vi "G#Debugger_OpenAttributeReference.vi"(0 "vi path":path, 5 "error in (no error)":errorcluster) -> (14 "vi reference":refnum<vi>, 19 "error out":errorcluster)   [LabVIEW 2017, in "G#Debugger.lvlib"]
uses:
  <vilib>/addons/_AddQ/G#Debugger/G#Debugger.lvlib
  <vilib>/Utility/miscctls.llb/LVPointTypeDef.ctl
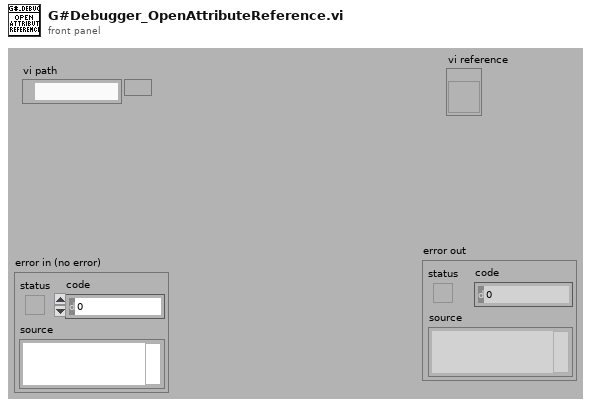
[diagram p1: front panel]
types:
  T1 = enum32{"invalid VI type", "Standard VI", "Control VI", "Global VI", "Polymorphic VI", "Configuration VI", "SubSystem", "Facade VI", "Method VI", "Statechart Diagram VI"}
  T2 = typedef "LVPointTypeDef.ctl" = cluster{"Horizontal":i16, "Vertical":i16}
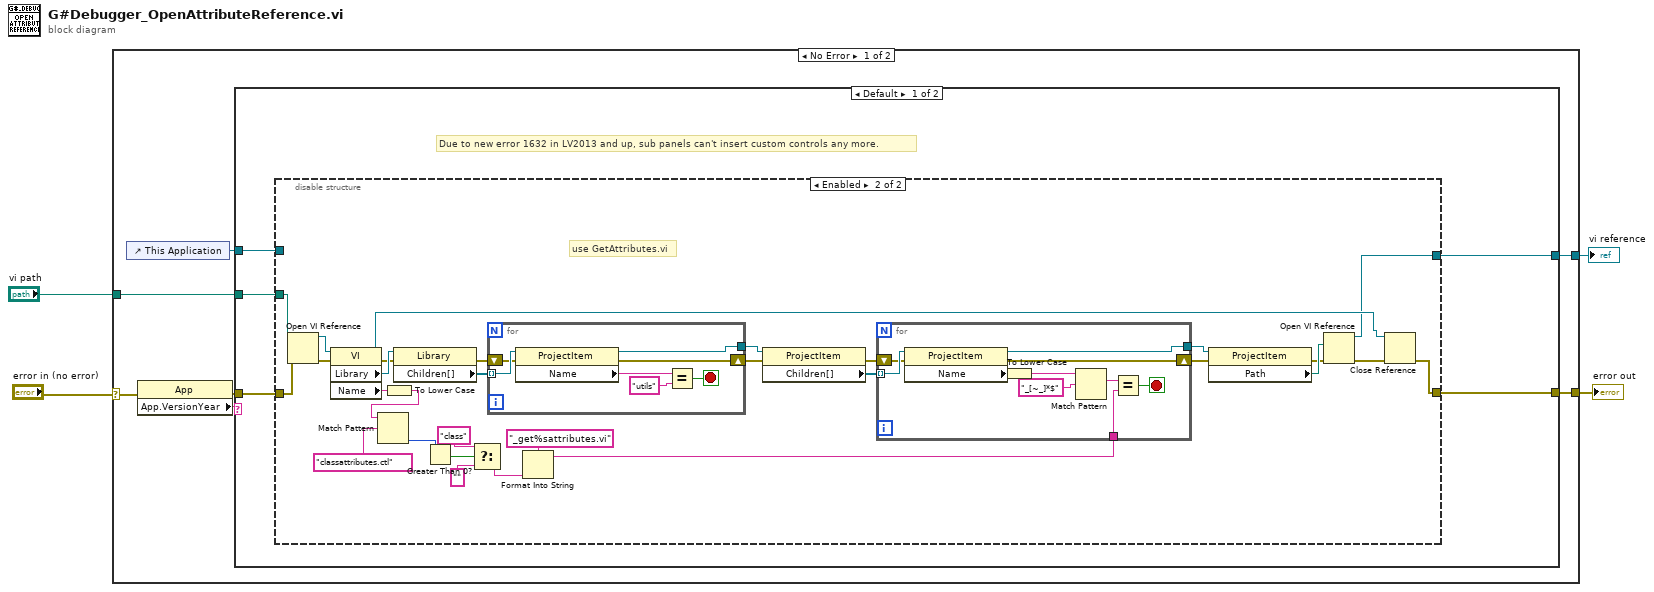
[diagram p0: block diagram]
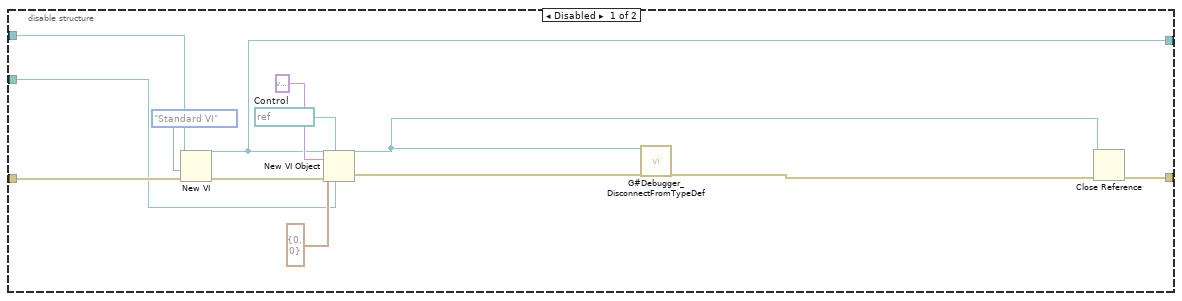
[diagram p2: hidden frame]
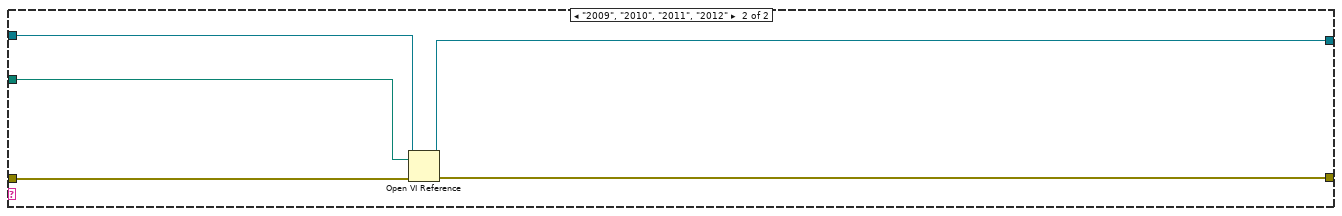
[diagram p3: hidden frame]
diagram:
  n1 = case shown="No Error" "error in (no error)" {
    selector: "error in (no error)" -> [w7 w82]
    tunnel: "vi path" -> [w9 _]
    tunnel: [w8 w82] -> w2
    tunnel: [w5 _] -> w3
    frame No Error {
      n2 = control-ref of="This Application"() -> (w6:refnum<vi>)
      n3 = property class="App"(error in=w7) -> (error out=w10:errorcluster, "App.VersionYear"=w11:string)  [unwired: 1 in, 1 out]
      n4 = case shown="Default" w11 {
        tunnel: w10 -> [w16 w81]
        tunnel: w9 -> [w14 w80]
        tunnel: [w15 w79] -> w8
        tunnel: w6 -> [w13 w78]
        tunnel: [w12 w77] -> w5
        frame Default {
          # "Due to new error 1632 in LV2013 and up, sub panels can't insert custom controls any more."
          n5 = disable-structure shown="Enabled" {
            disable-tunnel: w16 -> [w26 w45]
            disable-tunnel: [w25 w41] -> w15
            disable-tunnel: w14 -> [w24 w44]
            disable-tunnel: w13 -> [w22 _]
            disable-tunnel: [w20 w40] -> w12
            frame Disabled {
              w29 = refnum<vi> refnum  # Control
              n6 = New VI(8:w26, 9:T1."Standard VI" ("vi type (standard vi)"), 11:w22) -> (0:w23:errorcluster, 3:w20:refnum<vi>)  [unwired: 4 in]
              n7 = New VI Object(vi object class=w29, owner refnum=w20, style=variant, position/next to=T2 {"Horizontal"=0, "Vertical"=0} ("location"), 6:w24, 8:w23) -> (object refnum=w17:refnum<vi>, 0:w19:errorcluster)  [unwired: 2 in]
              n8 = call <vilib>:"G#Debugger_DisconnectFromTypeDef.vi"("Ctl Refnum"=w17, "error in (no error)"=w19) -> ("error out"=w18:errorcluster)  [unwired: 17 in]
              n9 = Close Reference(reference=w17, error in (no error)=w18) -> (error out=w25:errorcluster)
            }
            frame Enabled {
              # "use GetAttributes.vi"
              n10 = Open VI Reference(vi path=w44, error in (no error)=w45) -> (vi reference=w59:refnum<vi>, error out=w54:errorcluster)  [unwired: 4 in]
              n11 = property class="VI"(reference=w59, error in=w54) -> (reference out=w42:refnum<vi>, error out=w55:errorcluster, "Library"=w58:refnum<vi>, "Name"=w39:string)
              n12 = To Lower Case(string=w39) -> (all lower case string=w33:string)
              n13 = Match Pattern(string=w33, regular expression="classattributes.ctl") -> (offset past match=w31:i32)  [unwired: 1 in, 3 out]
              n14 = property class="Library"(reference=w58, error in=w55) -> (error out=w48:errorcluster, "Children[]"=w50:refnum<vi>[])  [unwired: 1 out]
              n15 = Greater Than 0?(x=w31) -> (x > 0?=w30:bool)
              n16 = Select(t="class" ("regular expression"), s=w30, f="" ("regular expression")) -> (s? t:f=w35:string)
              n17 = for {
                tunnel: w50 -> [w64] mode=indexing
                tunnel: [w62] -> w51
                shift-right: [w60] -> w47
                shift-left: w48 -> [w61]
                stop <- w63 stop-if-true
                n18 = property class="ProjectItem"(reference=w64, error in=w61) -> (reference out=w62:refnum<vi>, error out=w60:errorcluster, "Name"=w65:string)
                n19 = Equal?(x=w65, y="utils" ("regular expression")) -> (x = y?=w63:bool)
              }
              n20 = Format Into String(format string="_get%sattributes.vi" ("regular expression"), w35) -> (resulting string=w34:string)  [unwired: 2 in, 1 out]
              n21 = property class="ProjectItem"(reference=w51, error in=w47) -> (error out=w46:errorcluster, "Children[]"=w49:refnum<vi>[])  [unwired: 1 out]
              n22 = for {
                tunnel: w49 -> [w76] mode=indexing
                tunnel: [w72] -> w57
                shift-right: [w70] -> w53
                shift-left: w46 -> [w71]
                tunnel: w34 -> [w67]
                stop <- w73 stop-if-true
                n23 = property class="ProjectItem"(reference=w76, error in=w71) -> (reference out=w72:refnum<vi>, error out=w70:errorcluster, "Name"=w74:string)
                n24 = To Lower Case(string=w74) -> (all lower case string=w68:string)
                n25 = Match Pattern(string=w68, regular expression="_[~_]*$") -> (match substring=w69:string)  [unwired: 4 out]
                n26 = Equal?(x=w69, y=w67) -> (x = y?=w73:bool)
              }
              n27 = property class="ProjectItem"(reference=w57, error in=w53) -> (error out=w52:errorcluster, "Path"=w56:path)  [unwired: 1 out]
              n28 = Open VI Reference(vi path=w56, error in (no error)=w52) -> (vi reference=w40:refnum<vi>, error out=w43:errorcluster)  [unwired: 4 in]
              n29 = Close Reference(reference=w42, error in (no error)=w43) -> (error out=w41:errorcluster)
            }
          }
        }
        frame "2009", "2010", "2011", "2012" {
          n30 = Open VI Reference(application reference (local)=w78, vi path=w80, error in (no error)=w81) -> (vi reference=w77:refnum<vi>, error out=w79:errorcluster)  [unwired: 3 in]
        }
      }
    }
    frame Error {
    }
  }
  "vi reference" <- w3
  "error out" <- w2
